vi "tablaVerdad.vi"(9 "B":bool, 11 "A":bool) -> (3 "String":string)   [LabVIEW 2019, in "Prueba06.lvclass"]
uses:
  Prueba06.lvclass
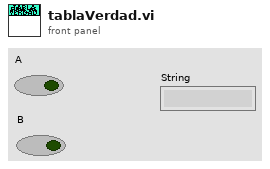
[diagram p1: front panel]
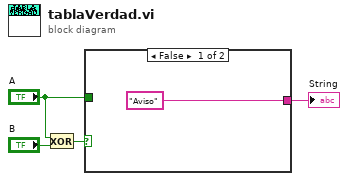
[diagram p0: block diagram]
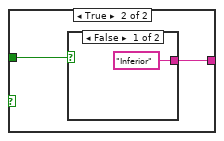
[diagram p2: hidden frame]
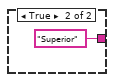
[diagram p3: hidden frame]
diagram:
  n1 = Exclusive Or(1:"B", 2:"A") -> (0:w3:bool)
  n2 = case shown="False" w3 {
    tunnel: "A" -> [_ w7]
    tunnel: ["Aviso" w6] -> w1
    frame False {
    }
    frame True {
      n3 = case shown="False" w7 {
        tunnel: ["Inferior" "Superior"] -> w6
        frame False {
        }
        frame True {
        }
      }
    }
  }
  "String" <- w1
